vi "SetupEQE_ActiveX.vi"(6 "Skip?":bool, 8 "error in (no error)":errorcluster) -> (0 "error out":errorcluster)   [LabVIEW 2016]
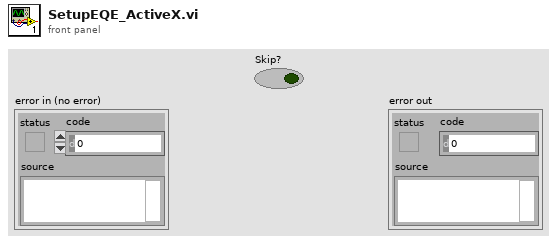
[diagram p1: front panel]
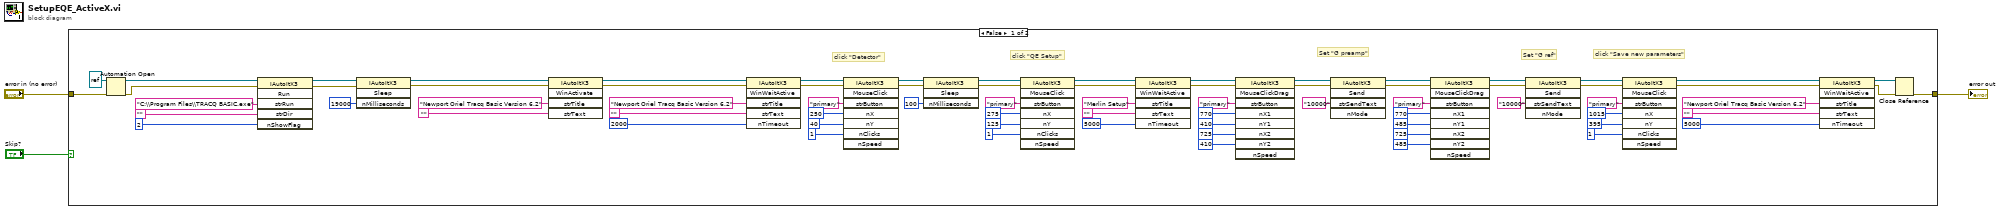
[diagram p0: block diagram]
diagram:
  n1 = case shown="False" "Skip?" {
    tunnel: "error in (no error)" -> [w7 w77]
    tunnel: [w74 w77] -> w2
    frame False {
      # "click \"Save new parameters\""
      # "Set \"G ref\""
      # "Set \"G preamp\""
      # "click \"QE Setup\""
      # "click \"Detector\""
      n2 = Automation Open(error in (no error)=w7, Automation Refnum=refnum<k7> refnum ("AutoItX3Lib.IAutoItX3")) -> (Automation Refnum=w11:refnum<k7>, error out=w10:errorcluster)  [unwired: 2 in]
      n3 = invoke class="IAutoItX3" method="Run"(reference=w11, error in=w10, "strRun"="C:\\Program Files\\TRACQ BASIC.exe", "strDir"="", "nShowFlag"=2) -> (reference out=w9:refnum<k7>, error out=w8:errorcluster)  [unwired: 1 in, 4 out]
      n4 = invoke class="IAutoItX3" method="Sleep"(reference=w9, error in=w8, "nMilliseconds"=19000) -> (reference out=w72:refnum<k7>, error out=w73:errorcluster)  [unwired: 1 in, 2 out]
      n5 = invoke class="IAutoItX3" method="WinActivate"(reference=w72, error in=w73, "strTitle"="Newport Oriel Tracq Basic Version 6.2", "strText"="") -> (reference out=w71:refnum<k7>, error out=w64:errorcluster)  [unwired: 1 in, 3 out]
      n6 = invoke class="IAutoItX3" method="WinWaitActive"(reference=w71, error in=w64, "strTitle"="Newport Oriel Tracq Basic Version 6.2", "strText"="", "nTimeout"=2000) -> (reference out=w65:refnum<k7>, error out=w63:errorcluster)  [unwired: 1 in, 4 out]
      n7 = invoke class="IAutoItX3" method="MouseClick"(reference=w65, error in=w63, "strButton"="primary", "nX"=250, "nY"=40, "nClicks"=1) -> (reference out=w57:refnum<k7>, error out=w56:errorcluster)  [unwired: 2 in, 6 out]
      n8 = invoke class="IAutoItX3" method="Sleep"(reference=w57, error in=w56, "nMilliseconds"=100) -> (reference out=w51:refnum<k7>, error out=w50:errorcluster)  [unwired: 1 in, 2 out]
      n9 = invoke class="IAutoItX3" method="MouseClick"(reference=w51, error in=w50, "strButton"="primary", "nX"=275, "nY"=125, "nClicks"=1) -> (reference out=w46:refnum<k7>, error out=w45:errorcluster)  [unwired: 2 in, 6 out]
      n10 = invoke class="IAutoItX3" method="WinWaitActive"(reference=w46, error in=w45, "strTitle"="Merlin Setup", "strText"="", "nTimeout"=5000) -> (reference out=w44:refnum<k7>, error out=w43:errorcluster)  [unwired: 1 in, 4 out]
      n11 = invoke class="IAutoItX3" method="MouseClickDrag"(reference=w44, error in=w43, "strButton"="primary", "nX1"=770 ("nX"), "nY1"=410 ("nY"), "nX2"=725 ("nClicks"), "nY2"=410 ("nClicks")) -> (reference out=w37:refnum<k7>, error out=w36:errorcluster)  [unwired: 2 in, 7 out]
      n12 = invoke class="IAutoItX3" method="Send"(reference=w37, error in=w36, "strSendText"="10000") -> (reference out=w26:refnum<k7>, error out=w25:errorcluster)  [unwired: 2 in, 3 out]
      n13 = invoke class="IAutoItX3" method="MouseClickDrag"(reference=w26, error in=w25, "strButton"="primary", "nX1"=770 ("nX"), "nY1"=485 ("nY"), "nX2"=725 ("nClicks"), "nY2"=485 ("nClicks")) -> (reference out=w29:refnum<k7>, error out=w28:errorcluster)  [unwired: 2 in, 7 out]
      n14 = invoke class="IAutoItX3" method="Send"(reference=w29, error in=w28, "strSendText"="10000") -> (reference out=w20:refnum<k7>, error out=w19:errorcluster)  [unwired: 2 in, 3 out]
      n15 = invoke class="IAutoItX3" method="MouseClick"(reference=w20, error in=w19, "strButton"="primary", "nX"=1015, "nY"=395, "nClicks"=1) -> (reference out=w15:refnum<k7>, error out=w14:errorcluster)  [unwired: 2 in, 6 out]
      n16 = invoke class="IAutoItX3" method="WinWaitActive"(reference=w15, error in=w14, "strTitle"="Newport Oriel Tracq Basic Version 6.2", "strText"="", "nTimeout"=5000) -> (reference out=w13:refnum<k7>, error out=w12:errorcluster)  [unwired: 1 in, 4 out]
      n17 = Close Reference(reference=w13, error in (no error)=w12) -> (error out=w74:errorcluster)
    }
    frame True {
    }
  }
  "error out" <- w2
